vi "Load EtherCAT Configuration.vi"() -> (2 "Map":T1(c390), 3 "ENI File":path)   [LabVIEW 2024, in "Hardware Controller.lvlib"]
uses:
  Hardware Controller.lvlib
  EtherCAT Configuration.ctl
  f90ee752-8a6c-4a81-ab6b-c1f334ecfc6f.vi
  <vilib>/JDP Science/JSONtext/JSON text to Variant.vi
  <vilib>/JDP Science/JSONtext/LVClass Serializer/JSONtext LVClass Serializer.lvclass
  <vilib>/JDP Science/JSONtext/Config Files/Config File.lvclass
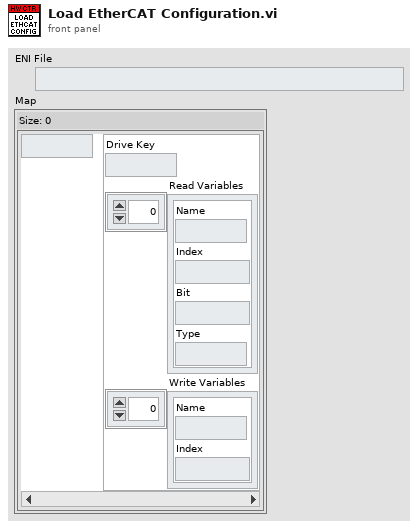
[diagram p1: front panel]
types:
  T1 = map{string, cluster{"Drive Key":string, "Read Variables":cluster{"Name":string, "Index":u16, "Bit":u8, "Type":string}[], "Write Variables":cluster{"Name":string, "Index":u16}[]}}
  T2 = typedef "EtherCAT Configuration.ctl" = cluster{"ENI File":path, "Drives":cluster{"Drive Key":string, "Read Variables":cluster{"Name":string, "Index":u16, "Bit":u8, "Type":string}[], "Write Variables":cluster{"Name":string, "Index":u16}[]}[]}
  T3 = cluster{"Drive Key":string, "Read Variables":cluster{"Name":string, "Index":u16, "Bit":u8, "Type":string}[], "Write Variables":cluster{"Name":string, "Index":u16}[]}[]
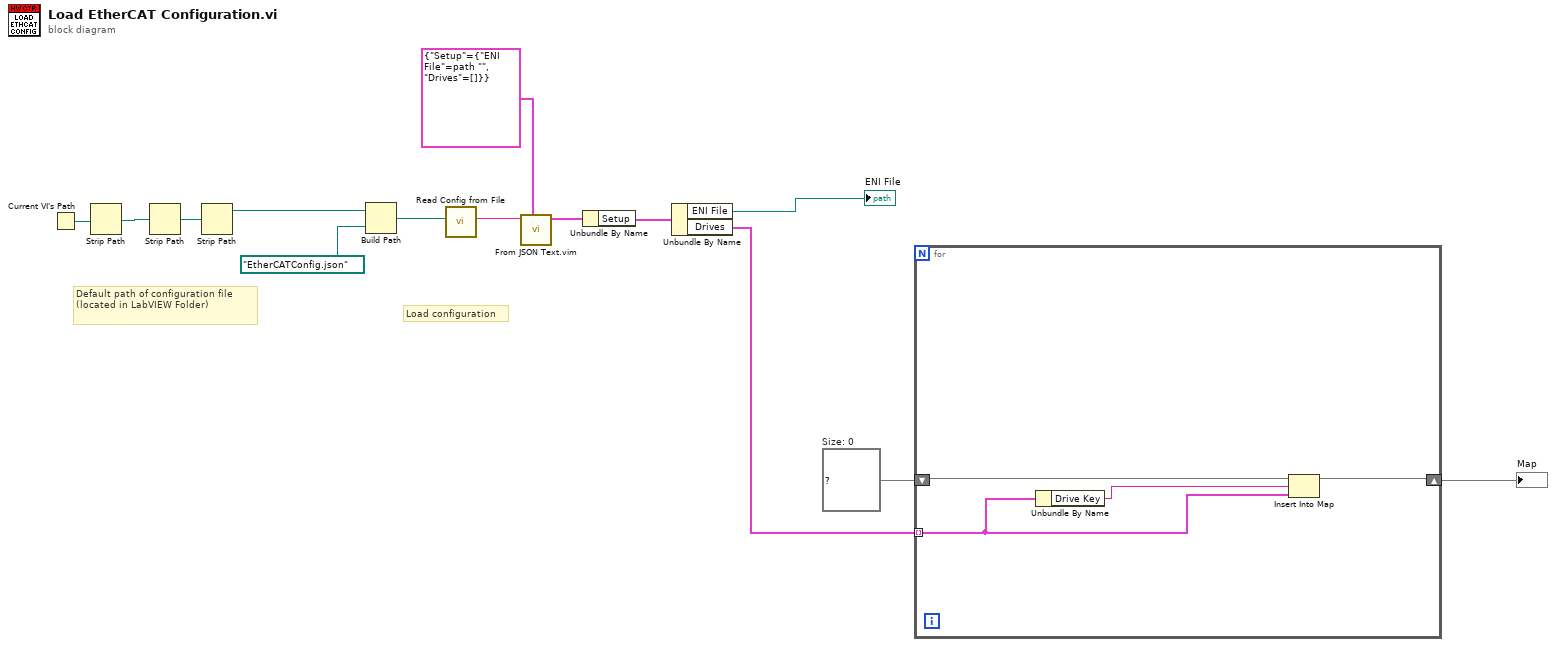
[diagram p0: block diagram]
diagram:
  w2 = T1 {}  # Size: 0
  # "Load configuration"
  # "Default path of configuration file (located in LabVIEW Folder)"
  n1 = Current VI's Path() -> (path=w14:path)
  n2 = Strip Path(path=w14) -> (stripped path=w13:path)  [unwired: 1 out]
  n3 = Strip Path(path=w13) -> (stripped path=w11:path)  [unwired: 1 out]
  n4 = Strip Path(path=w11) -> (stripped path=w10:path)  [unwired: 1 out]
  n5 = Build Path(base path=w10, name or relative path=path "EtherCATConfig.json") -> (appended path=w8:path)
  n6 = call <vilib>:"Read Config from File.vi"("config file path"=w8) -> ("<JSON>Config"=w9:string)  [unwired: 7 in, 3 out]
  n7 = call "From JSON Text.vim"("Data Type and Default Value"=cluster{"Setup":T2} {"Setup"={"ENI File"=path "", "Drives"=[]}}, "JSON"=w9) -> ("Data out"=w6:cluster{"Setup":T2})  [unwired: 8 in, 1 out]
  n8 = Unbundle By Name(w6) -> ("Setup"=w5:T2)
  n9 = Unbundle By Name(w5) -> ("ENI File"=→"ENI File":path, "Drives"=w3:T3)
  n10 = for {
    tunnel: w3 -> [w15] mode=indexing
    shift-right: [w18] -> w1
    shift-left: w2 -> [w17]
    n11 = Unbundle By Name(w15) -> ("Drive Key"=w16:string)
    n12 = Insert Into Map(map in=w17, key=w16, value=w15) -> (map out=w18:T1)  [unwired: 2 out]
  }
  "Map" <- w1
